vi "Find Aircraft UDP Port.vi"(8 "Error In":errorcluster) -> (0 "Error Out":errorcluster, 3 "UDP Ref Out":refnum<k16>)   [LabVIEW 2014]
panel:
  out "IP Address":string
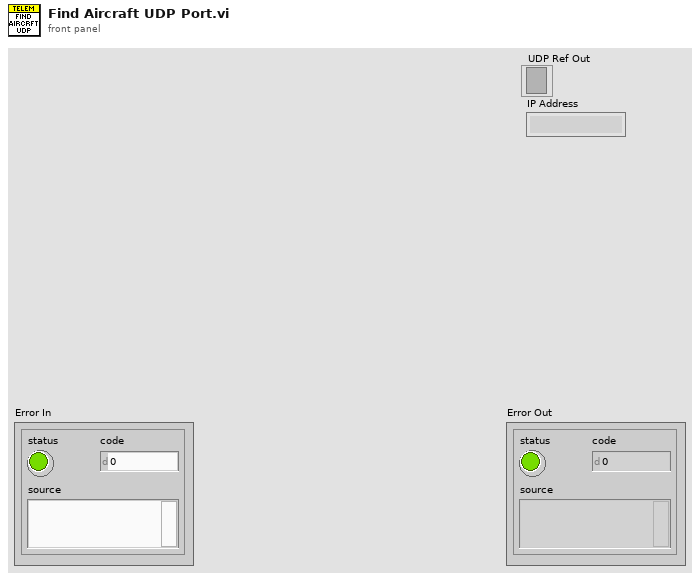
[diagram p1: front panel]
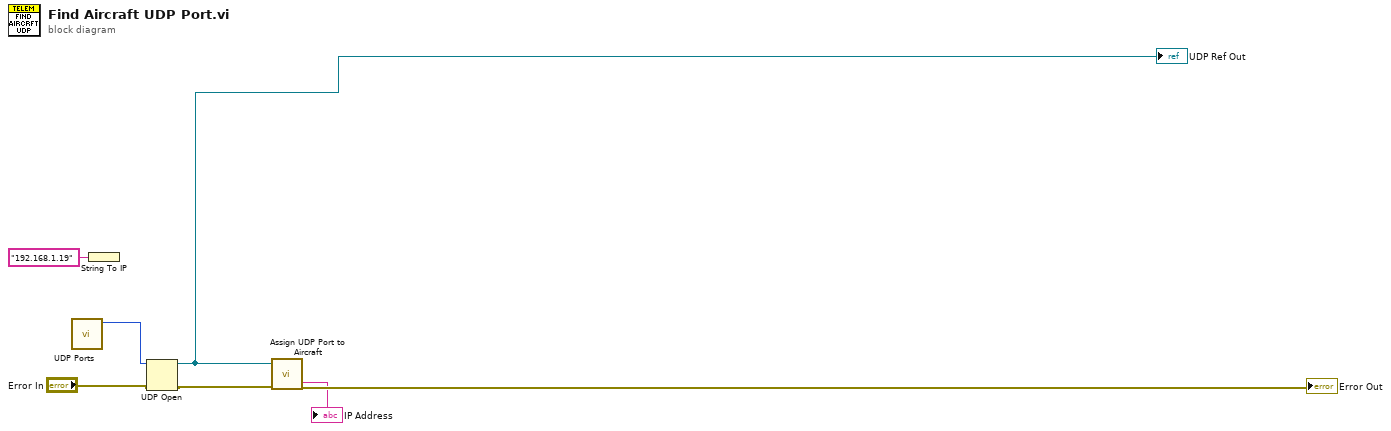
[diagram p0: block diagram]
diagram:
  n1 = call "UDP Ports.vi"() -> ("RX Port"=w4:u16)  [unwired: 9 in, 2 out]
  n2 = String To IP(1:"192.168.1.19" ("name")) -> ()  [unwired: 1 out]
  n3 = UDP Open(8:"Error In", 11:w4) -> (port=w1:refnum<k16>, 0:w6:errorcluster)  [unwired: 3 in, 1 out]
  "UDP Ref Out" <- w1
  n4 = call "Assign UDP Port to Aircraft.vi"("error out"=w6, "UDP Port Ref"=w1) -> ("error out"=→"Error Out":errorcluster, "IP Address"=→"IP Address":string)  [unwired: 5 in, 3 out]
